vi "REF Array Add or Remove.vi"(8 "error in (no error)":errorcluster, 11 "REF Channels in":T1=[{"Enable?"=FALSE, "Channel"=13, "Frequency"=0.1, "Phase"=0.0, "TC"=1e-05, "Roll-Off"=1}] {"Roll-Off" min=1; "TC" min=0.0001 format="%#_3p"; "Phase" format="%.3g"; "Frequency" min=0.0001 max=10000.0 format="%.3g"}) -> (0 "error out":errorcluster, 3 "REF Channels out":T1=[{"Enable?"=FALSE, "Channel"=13, "Frequency"=0.1, "Phase"=0.0, "TC"=1e-05, "Roll-Off"=1}] {"Roll-Off" min=1; "TC" min=0.0001 format="%#_3p"; "Phase" format="%.3g"; "Frequency" min=0.0001 max=10000.0 format="%.3g"})   [LabVIEW 2019, in "Instrument.Lockin.lvclass"]
uses:
  Instrument.Lockin.lvclass
  Instrument.DAQ/Typedefs/REF-cluster.ctl
  Instrument UI.Lockin/Typedefs/REF Channel--Cluster.ctl
  Instrument UI.Lockin/Instrument UI.Lockin.lvclass
  Instrument.DAQ/Instrument.DAQ.lvclass
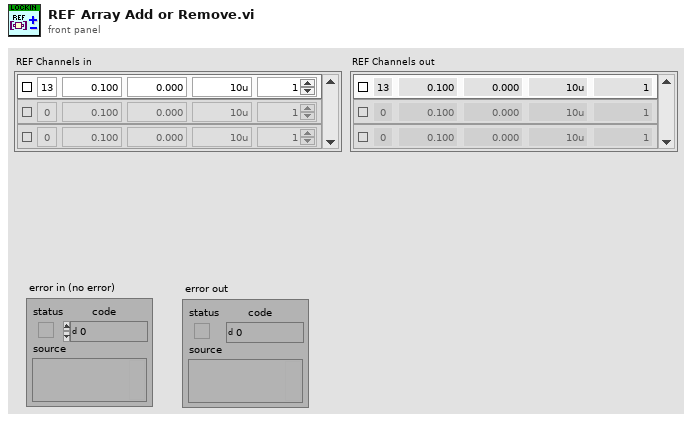
[diagram p1: front panel]
types:
  T1 = typedef "Instrument.DAQ.lvclass/REF-cluster.ctl" = T2[]
  T2 = typedef "Instrument UI.Lockin.lvclass/REF Channel--Cluster.ctl" = cluster{"Enable?":bool, "Channel":i32, "Frequency":dbl, "Phase":dbl, "TC":dbl, "Roll-Off":i32}
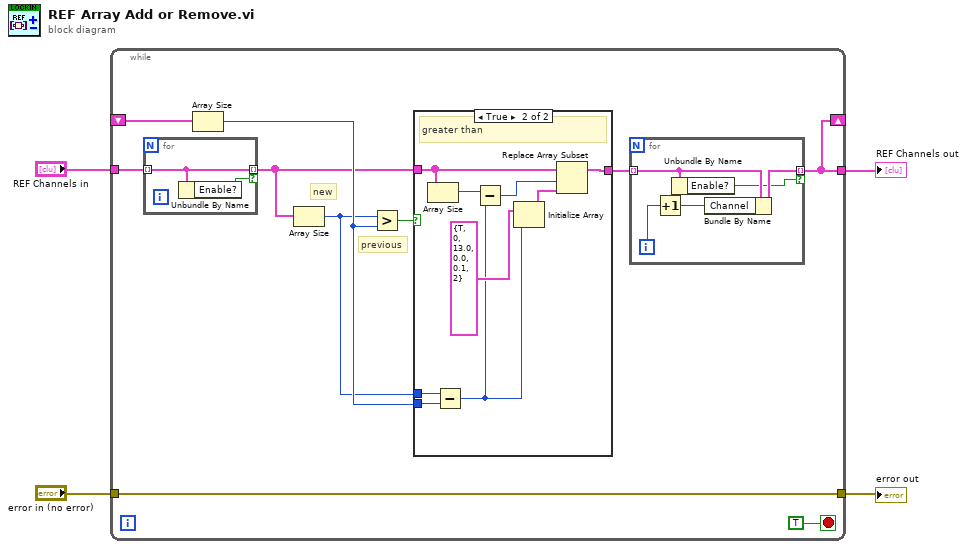
[diagram p0: block diagram]
diagram:
  n1 = while {
    tunnel: "REF Channels in" -> [w6]
    tunnel: [w10] -> w3
    tunnel: "error in (no error)" -> [w12]
    tunnel: [w12] -> w1
    shift-right: [w10] -> _
    shift-left: _ -> [w9]
    stop <- TRUE stop-if-true
    # "new"
    # "previous"
    n2 = for {
      tunnel: w6 -> [w15] mode=indexing
      tunnel: [w15] -> w5 mode=indexing if=w16
      n3 = Unbundle By Name(w15) -> ("Enable?"=w16:bool)
    }
    n4 = Array Size(array=w9) -> (size(s)=w8:i32)
    n5 = Array Size(array=w5) -> (size(s)=w7:i32)
    n6 = Greater?(x=w7, y=w8) -> (0:w14:bool)
    n7 = case shown="True" w14 {
      tunnel: w5 -> [w22 w26]
      tunnel: w7 -> [_ w31]
      tunnel: [w22 w27] -> w13
      tunnel: w8 -> [_ w30]
      frame False {
        # "less than or equal"
      }
      frame True {
        # "greater than"
        n8 = Array Size(array=w26) -> (size(s)=w25:i32)
        n9 = Subtract(x=w31, y=w30) -> (x-y=w24:i32)
        n10 = Subtract(x=w25, y=w24) -> (x-y=w23:i32)
        n11 = Initialize Array(T2 {"Enable?"=TRUE, "Channel"=0, "Frequency"=13.0, "Phase"=0.0, "TC"=0.1, "Roll-Off"=2} ("REF"), w24) -> (w28:T2[])
        n12 = Replace Array Subset(array=w26, new element=w28, index=w23) -> (w27:T2[])
      }
    }
    n13 = for {
      tunnel: w13 -> [w18] mode=indexing
      tunnel: [w21] -> w10 mode=indexing if=w17
      i -> [w19]
      n14 = Increment(x=w19) -> (x+1=w20:i32)
      n15 = Unbundle By Name(w18) -> ("Enable?"=w17:bool)
      n16 = Bundle By Name(cluster=w18, "Channel"=w20) -> (w21:T2)
    }
  }
  "REF Channels out" <- w3
  "error out" <- w1
